vi "19-MatchAxis.vi"(7 "Axis":enum16{"x", "y", "z"}(ring), 9 "Minimum Matches":i32, 10 "Base Sensor Orientation Info":T1, 11 "Orientation Info":T1) -> (2 "Match Translations":i32[](array[numeric]), 3 "Matches":cluster{"Beacons":i32[][]}[](array[cluster]))   [LabVIEW 2019, in "19.lvlib"]
uses:
  19.lvlib
  92d0060c-6fae-4986-a4ac-6404e40ef244.vi
  <vilib>/Array/Sort 2D Array - Pop Stack.vi
  <vilib>/Array/Sort 2D Array - Push Stack.vi
  92d0060c-6fae-4986-a4ac-6404e40ef244.vi/534957bd-c714-43cc-a3be-7c7abc716df5.vi
  92d0060c-6fae-4986-a4ac-6404e40ef244.vi/0b6f0fae-ad62-49f3-a759-33a91d28884f.vi
  <userlib>/_OpenG.lib/array/array.llb/Search 1D Array (I32)__ogtk.vi
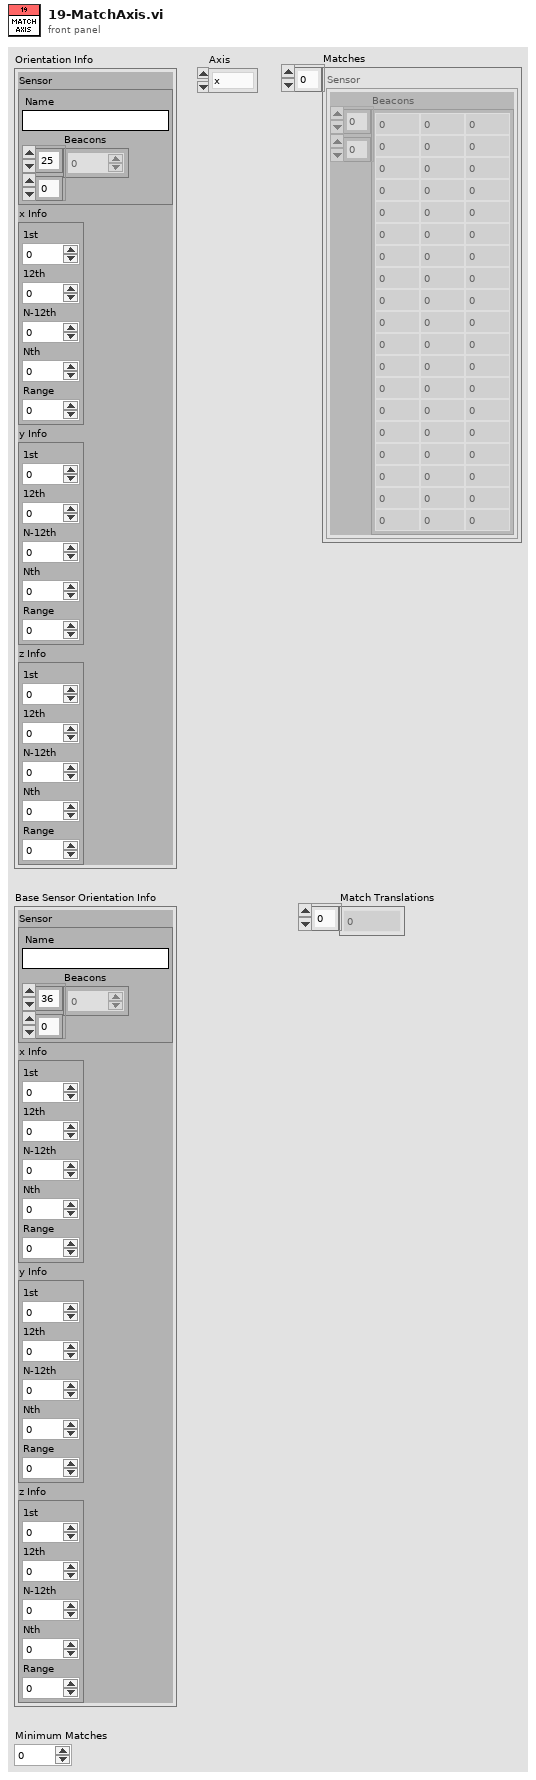
[diagram p1: front panel]
types:
  T1 = cluster{"Sensor":cluster{"Name":string, "Beacons":i32[][]}, "x Info":cluster{"1st":i32, "12th":i32, "N-12th":i32, "Nth":i32, "Range":i32}, "y Info":cluster{"1st":i32, "12th":i32, "N-12th":i32, "Nth":i32, "Range":i32}, "z Info":cluster{"1st":i32, "12th":i32, "N-12th":i32, "Nth":i32, "Range":i32}}
  T2 = cluster{"1st":i32, "12th":i32, "N-12th":i32, "Nth":i32, "Range":i32}
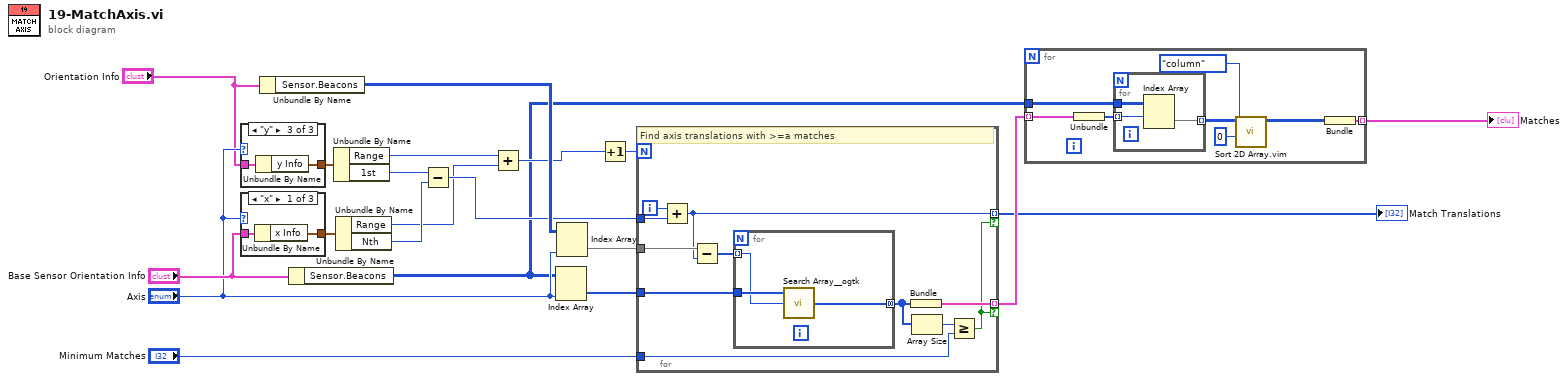
[diagram p0: block diagram]
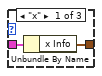
[diagram p2: hidden frame]
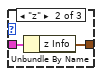
[diagram p3: hidden frame]
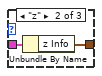
[diagram p4: hidden frame]
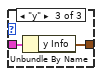
[diagram p5: hidden frame]
diagram:
  n1 = case shown="\"y\"" "Axis" {
    tunnel: "Orientation Info" -> [w22 w24 w26]
    tunnel: [w21 w23 w25] -> w17
    frame "x" {
      n2 = Unbundle By Name(w22) -> ("x Info"=w21:T2)
    }
    frame "z" {
      n3 = Unbundle By Name(w24) -> ("z Info"=w23:T2)
    }
    frame "y" {
      n4 = Unbundle By Name(w26) -> ("y Info"=w25:T2)
    }
  }
  n5 = case shown="\"x\"" "Axis" {
    tunnel: "Base Sensor Orientation Info" -> [w28 w30 w32]
    tunnel: [w27 w29 w31] -> w18
    frame "x" {
      n6 = Unbundle By Name(w28) -> ("x Info"=w27:T2)
    }
    frame "z" {
      n7 = Unbundle By Name(w30) -> ("z Info"=w29:T2)
    }
    frame "y" {
      n8 = Unbundle By Name(w32) -> ("y Info"=w31:T2)
    }
  }
  n9 = Unbundle By Name("Orientation Info") -> ("Sensor.Beacons"=w15:i32[][])
  n10 = Unbundle By Name("Base Sensor Orientation Info") -> ("Sensor.Beacons"=w3:i32[][])
  n11 = Unbundle By Name(w17) -> ("Range"=w7:i32, "1st"=w10:i32)
  n12 = Unbundle By Name(w18) -> ("Range"=w6:i32, "Nth"=w9:i32)
  n13 = Subtract(x=w10, y=w9) -> (x-y=w8:i32)
  n14 = Add(x=w7, y=w6) -> (x+y=w5:i32)
  n15 = Index Array(array=w3, index (col)="Axis") -> (element=w1:i32[])  [unwired: 1 in]
  n16 = Index Array(array=w15, index (col)="Axis") -> (element=w2:i32[])  [unwired: 1 in]
  n17 = Increment(x=w5) -> (x+1=w11:i32)
  n18 = for {
    N: w11 -> [_]
    tunnel: w2 -> [w43]
    tunnel: w1 -> [w33]
    tunnel: [w40] -> w16 mode=indexing if=w39
    tunnel: "Minimum Matches" -> [w41]
    tunnel: [w36] -> w13 mode=indexing if=w39
    tunnel: w8 -> [w37]
    i -> [w38]
    # "Find axis translations with >=a matches"
    n19 = Add(x=w38, y=w37) -> (x+y=w36:i32)
    n20 = Subtract(x=w43, y=w36) -> (x-y=w34:i32[])
    n21 = for {
      tunnel: w33 -> [w46]
      tunnel: w34 -> [w45] mode=indexing
      tunnel: [w44] -> w42 mode=concatenating
      n22 = call-poly <userlib>:"Search Array__ogtk.vi"("Array"=w46, "Element Data"=w45) -> ("Indices of Elements"=w44:i32[])  [unwired: 7 in]
    }
    n23 = Bundle("Indices of Elements"=w42) -> (w40:cluster{"Indices of Elements":i32[]})  [unwired: 1 in]
    n24 = Array Size(array=w42) -> (size(s)=w35:i32)
    n25 = Greater Or Equal?(x=w35, y=w41) -> (x >= y?=w39:bool)
  }
  "Match Translations" <- w13
  n26 = for {
    tunnel: w16 -> [w54] mode=indexing
    tunnel: w3 -> [w52]
    tunnel: [w50] -> w14 mode=indexing
    n27 = Unbundle(w54) -> ("Indices of Elements"=w53:i32[])
    n28 = for {
      tunnel: w53 -> [w56] mode=indexing
      tunnel: w52 -> [w57]
      tunnel: [w55] -> w51 mode=indexing
      n29 = Index Array(array=w57, index (row)=w56) -> (element=w55:i32[])  [unwired: 1 in]
    }
    n30 = call "Sort 2D Array.vim"("index"=0, "dimension to index (column)"=enum16{"column", "row"}."column", "2D array"=w51) -> ("sorted 2D array"=w49:i32[][])  [unwired: 7 in, 1 out]
    n31 = Bundle("sorted 2D array"=w49) -> (w50:cluster{"sorted 2D array":i32[][]})  [unwired: 1 in]
  }
  "Matches" <- w14
